vi "Read Class Type.vi"(8 "error in (no error)":errorcluster, 11 "IC.lvclass in":refnum<class "NI_IC.lvclass">) -> (0 "error out":errorcluster, 2 "IC class type":T1 items=["IC"=0, "IC_1D"=10, "IC_1D_Numeric"=11, "IC_1D_VIRef"=12, "IC_2D"=20, "IC_2D_Numeric"=21, "IC_2D_VIRef"=22], 3 "IC.lvclass out":refnum<class "NI_IC.lvclass">)   [LabVIEW 2020, in "NI_PDE.lvlib" / "NI_IC.lvclass"]
uses:
  <vilib>/gmath/pde.llb/ICClass/NI_IC.lvclass
  <vilib>/gmath/pde.llb/ICClass/Class Type.ctl
  <vilib>/gmath/pde.llb/ICClass/NI_IC.lvclass/NI_IC.ctl
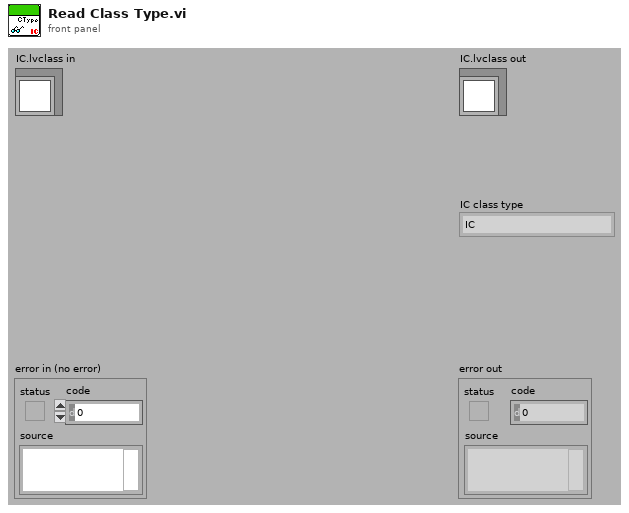
[diagram p1: front panel]
types:
  T1 = typedef "NI_PDE.lvlib/NI_IC.lvclass/Class Type.ctl" = i32
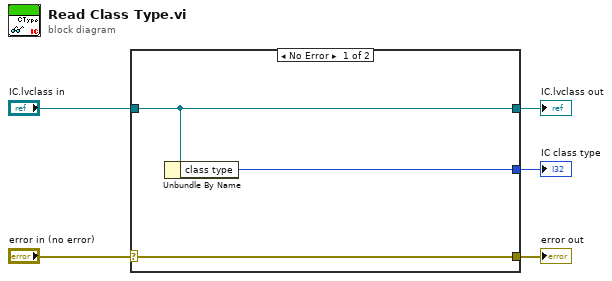
[diagram p0: block diagram]
diagram:
  n1 = case shown="No Error" "error in (no error)" {
    selector: "error in (no error)" -> [w8 w9]
    tunnel: [w8 w9] -> w4
    tunnel: [w7 w10] -> w2
    tunnel: "IC.lvclass in" -> [w7 w10]
    tunnel: [w6 _] -> w1
    frame No Error {
      n2 = Unbundle By Name(w7) -> ("class type"=w6:T1)
    }
    frame Error {
    }
  }
  "error out" <- w4
  "IC.lvclass out" <- w2
  "IC class type" <- w1
